vi "zad6.vi"() -> ()   [LabVIEW 2023]
panel:
  out "XY Graph":cluster{u32[], dbl[]}[](graph)
  out "error out":errorcluster
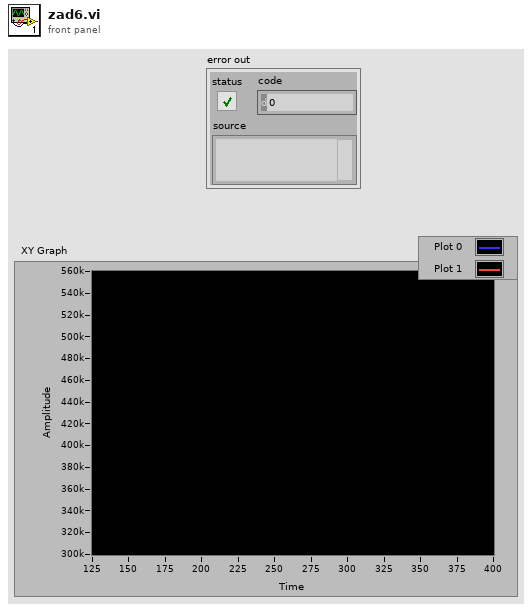
[diagram p1: front panel]
types:
  T1 = enum16{"open", "replace", "create", "open or create", "replace or create", "replace or create with confirmation"}
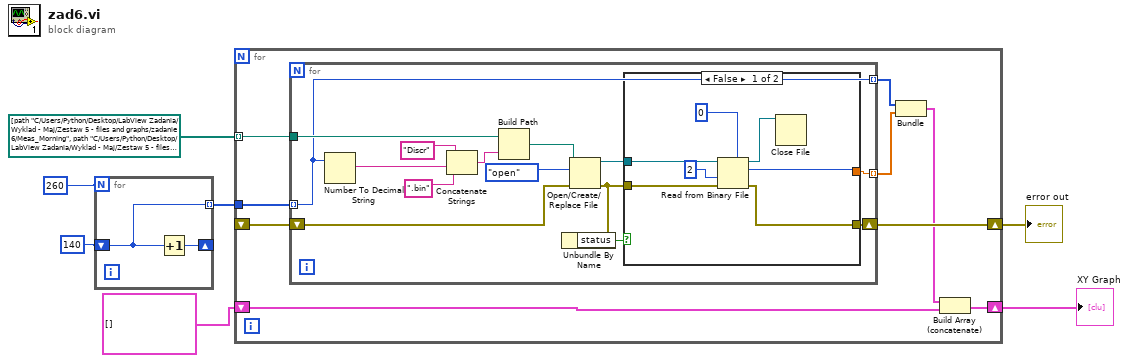
[diagram p0: block diagram]
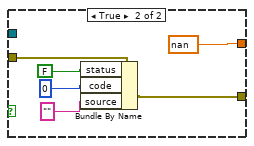
[diagram p2: hidden frame]
diagram:
  n1 = for {
    N: 260 -> [_]
    shift-right: [w9] -> _
    shift-left: 140 -> [w8]
    tunnel: [w8] -> w4 mode=indexing
    n2 = Increment(x=w8) -> (x+1=w9:i32)
  }
  n3 = for {
    tunnel: path[] [path "C:/Users/Python/Desktop/LabView Zadania/Wyklad - Maj/Zestaw 5 - files and graphs/zadanie 6/Meas_Morning", path "C:/Users/Python/Desktop/LabView Zadania/Wyklad - Maj/Zestaw 5 - files and graphs/zadanie 6/Meas_Evening"] ("Array") -> [w18] mode=indexing
    tunnel: w4 -> [w17]
    shift-right: [w16] -> w3
    shift-left: _ -> [w15]
    shift-right: [w11] -> w1
    shift-left: cluster{u32[], u32[]}[] [] -> [w12]
    n4 = for {
      tunnel: w18 -> [w32]
      tunnel: w17 -> [w21] mode=indexing
      shift-right: [w23] -> w16
      shift-left: w15 -> [w22]
      tunnel: [w21] -> w14 mode=indexing
      tunnel: [w20] -> w13 mode=indexing
      n5 = Number To Decimal String(number=w21) -> (decimal integer string=w28:string)  [unwired: 1 in]
      n6 = Concatenate Strings("Discr" ("string"), w28, ".bin" ("string")) -> (w31:string)
      n7 = Build Path(base path=w32, name or relative path=w31) -> (appended path=w27:path)
      n8 = Open/Create/Replace File(file path (use dialog)=w27, error in=w22, operation (0:open)=T1."open") -> (refnum out=w19:refnum<file>, error out=w24:errorcluster)  [unwired: 3 in, 1 out]
      n9 = Unbundle By Name(w24) -> ("status"=w25:bool)
      n10 = case shown="False" w25 {
        tunnel: w24 -> [w37 w45]
        tunnel: [w36 w41] -> w23
        tunnel: [w33 nan] -> w20
        tunnel: w19 -> [w39 _]
        frame False {
          n11 = Read from Binary File(5:u32 0, 8:w37, 9:2 ("count (1)"), 11:w39) -> (0:w36:errorcluster, 2:w33:u32, 3:w38:refnum<file>)  [unwired: 2 in, 1 out]
          n12 = Close File(refnum=w38) -> ()  [unwired: 1 in, 2 out]
        }
        frame True {
          n13 = Bundle By Name(cluster=w45, "status"=FALSE, "code"=0, "source"="") -> (w41:errorcluster)
        }
      }
    }
    n14 = Bundle(w14, w13) -> (w10:cluster{i32[], dbl[]})  [unwired: 1 in]
    n15 = Build Array (concatenate)(w10, w12) -> (w11:cluster{u32[], dbl[]}[])
  }
  "error out" <- w3
  "XY Graph" <- w1
